vi "ReplyToString.vi"(0 "Reply":T1, 11 "Error In":errorcluster) -> (4 "String":string, 15 "Error Out":errorcluster)   [LabVIEW 2020, in "Redis.lvclass"]
doc: "Converts the reply data to a string"
uses:
  Redis.lvclass
  RedisDataType.ctl
  ReplyDataTypeEnum.ctl
  Redis.lvclass/Redis.ctl
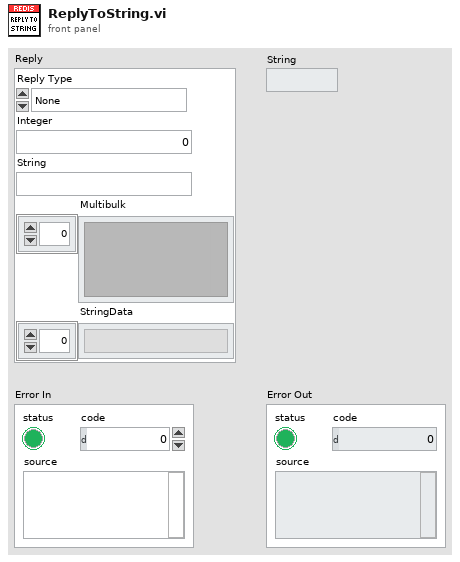
[diagram p1: front panel]
types:
  T1 = typedef "Redis.lvclass/RedisDataType.ctl" = cluster{"Reply Type":T2, "Integer":i64, "String":string, "Multibulk":variant[], "StringData":string[]}
  T2 = typedef "Redis.lvclass/ReplyDataTypeEnum.ctl" = enum16{"None", "Error", "Status", "Nil", "Integer", "String", "Multibulk"}
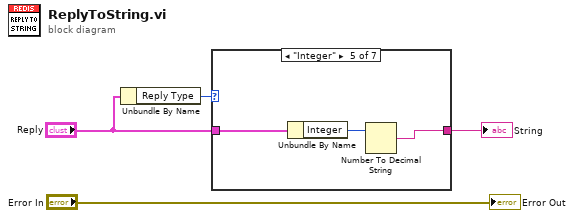
[diagram p0: block diagram]
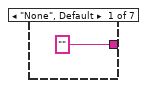
[diagram p2: hidden frame]
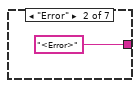
[diagram p3: hidden frame]
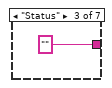
[diagram p4: hidden frame]
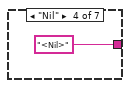
[diagram p5: hidden frame]
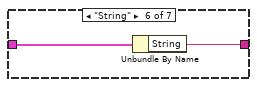
[diagram p6: hidden frame]
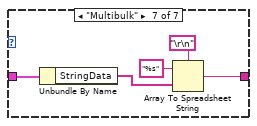
[diagram p7: hidden frame]
diagram:
  n1 = Unbundle By Name("Reply") -> ("Reply Type"=w2:T2)
  n2 = case shown="\"Integer\"" w2 {
    tunnel: "Reply" -> [_ _ _ _ w11 w13 w18]
    tunnel: ["" ("String") "<Error>" ("String") "" ("String") "<Nil>" ("String") w9 w12 w15] -> w3
    frame "None", Default {
    }
    frame "Error" {
    }
    frame "Status" {
    }
    frame "Nil" {
    }
    frame "Integer" {
      n3 = Unbundle By Name(w11) -> ("Integer"=w10:i64)
      n4 = Number To Decimal String(number=w10) -> (decimal integer string=w9:string)  [unwired: 1 in]
    }
    frame "String" {
      n5 = Unbundle By Name(w13) -> ("String"=w12:string)
    }
    frame "Multibulk" {
      n6 = Unbundle By Name(w18) -> ("StringData"=w17:string[])
      n7 = Array To Spreadsheet String(delimiter (Tab)="\r\n", array=w17, 3:"%s" ("format string")) -> (spreadsheet string=w15:string)
    }
  }
  "String" <- w3
  "Error Out" <- "Error In"
